vi "Stoic_Mean_Calc-Test.vi"() -> ()   [LabVIEW 2014]
uses:
  <vilib>/Analysis/baseanly.llb/Mean (DBL).vi
  <vilib>/Utility/file.llb/Read From Spreadsheet File (DBL).vi
  <vilib>/Analysis/NI_AALBase.lvlib
panel:
  out "Max":dbl format="%0.2f"
  out "Max Array":dbl[](array[numeric])
  in  "Test Vi":bool
  out "Mean":dbl format="%0.2f"
  out "Mean Array":dbl[](array[numeric])
  out "Min value":dbl
  out "Max value":dbl
  in  "Cycle Length":dbl
  out "20% Bin Index":i32[](array[numeric])
  out "Bin Array":dbl[](array[numeric])
  out "Temp Values":dbl[](array[numeric])
  in  "file path (dialog if empty)":path
  out "Max Bin":dbl
  out "Min Bin":dbl
  in  "Multiple":dbl
  in  "Array In":dbl[](array[numeric])
  # "Stoic Temperature Mean"
  # "Overall"
  # "Stoic"
  # "(Used for Testing)"
  # "For Testing VI:\nUse Tab delimited file from excel with all data Transposed\nto the top Row.\nOpen Vi in Windows not RT."
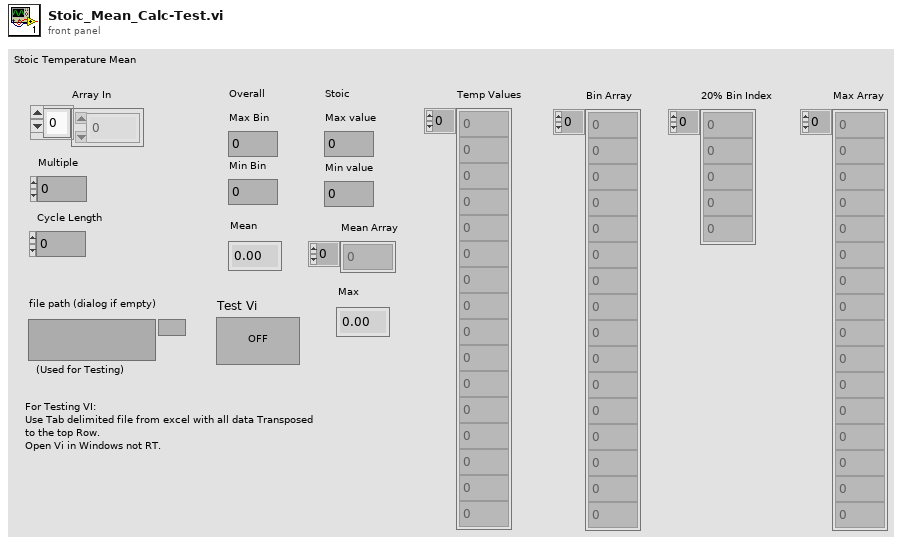
[diagram p1: front panel]
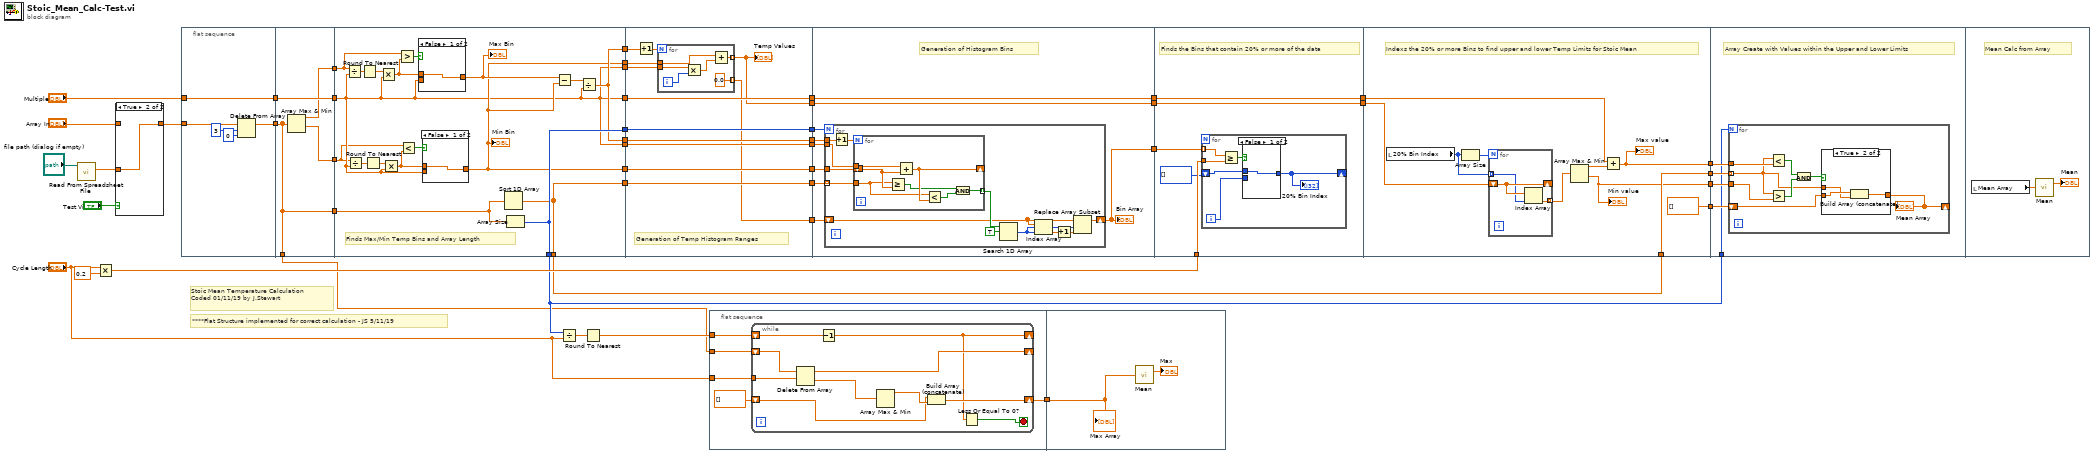
[diagram p0: block diagram]
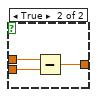
[diagram p3: hidden frame]
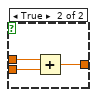
[diagram p4: hidden frame]
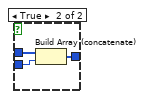
[diagram p5: hidden frame]
diagram:
  # "****Flat Structure implemented for correct calculation - JS 5/11/19"
  # "Stoic Mean Temperature Calculation\nCoded 01/11/19 by J.Stewart"
  n1 = call-poly <vilib>:"Read From Spreadsheet File.vi"("file path (dialog if empty)"="file path (dialog if empty)") -> ("first row"=w45:dbl[])  [unwired: 6 in, 4 out]
  n2 = Multiply(x="Cycle Length", y=0.2) -> (x*y=w38:dbl)
  n3 = case shown="True" "Test Vi" {
    tunnel: w45 -> [_ w49]
    tunnel: [w48 w49] -> w7
    tunnel: "Array In" -> [w48 _]
    frame False {
    }
    frame True {
    }
  }
  n4 = flat-sequence {
    tunnel: "Multiple" -> [w54]
    tunnel: [w54] -> w9
    tunnel: [w51] -> w8
    tunnel: w7 -> [w50]
    tunnel: [w58] -> w13
    tunnel: [w55] -> w12
    tunnel: [w57] -> w11
    tunnel: [w56] -> w10
    tunnel: w9 -> [w58]
    tunnel: w8 -> [w55]
    tunnel: [w55] -> w1
    tunnel: [w74] -> w23
    tunnel: [w65] -> w22
    tunnel: [w60] -> w21
    tunnel: [w73] -> w20
    tunnel: [w75] -> w19
    tunnel: [w60] -> w18
    tunnel: [w73] -> w17
    tunnel: [w65] -> w16
    tunnel: [w75] -> w3
    tunnel: [w74] -> w15
    tunnel: [w60] -> w14
    tunnel: w13 -> [w60]
    tunnel: w12 -> [w76]
    tunnel: w11 -> [w66]
    tunnel: w10 -> [w59]
    tunnel: [w89] -> w36
    tunnel: [w96] -> w35
    tunnel: [w95] -> w34
    tunnel: [w94] -> w33
    tunnel: [w93] -> w32
    tunnel: [w92] -> w31
    tunnel: [w85] -> w29
    tunnel: [w91] -> w26
    tunnel: w23 -> [w96]
    tunnel: w22 -> [w95]
    tunnel: w21 -> [w94]
    tunnel: w20 -> [w93]
    tunnel: w19 -> [w92]
    tunnel: w18 -> [w91]
    tunnel: w17 -> [w88]
    tunnel: w16 -> [w86]
    tunnel: w14 -> [w87]
    tunnel: [w111] -> w37
    tunnel: w36 -> [w110]
    tunnel: w35 -> [w109]
    tunnel: w34 -> [w108]
    tunnel: w33 -> [w107]
    tunnel: w32 -> [w106]
    tunnel: w31 -> [w105]
    tunnel: w29 -> [w104]
    tunnel: [w104] -> w28
    tunnel: w26 -> [w103]
    tunnel: [w103] -> w25
    tunnel: w38 -> [w134]
    tunnel: w37 -> [w135]
    tunnel: [w132] -> w30
    tunnel: w28 -> [w132]
    tunnel: [w131] -> w27
    tunnel: w25 -> [w131]
    tunnel: w15 -> [w155]
    tunnel: [w150] -> w42
    tunnel: [dbl[] [] ("Array 3")] -> w41
    tunnel: [w155] -> w40
    tunnel: [w149] -> w39
    tunnel: w30 -> [w147]
    tunnel: w27 -> [w146]
    tunnel: w42 -> [w162]
    tunnel: w41 -> [w161]
    tunnel: w40 -> [w160]
    tunnel: w39 -> [w163]
    tunnel: w3 -> [w159]
    frame #0 {
      n5 = Delete From Array(array=w50, length=3, index=0) -> (array with subset deleted=w51:dbl[])  [unwired: 1 out]
    }
    frame #1 {
      n6 = Array Max & Min(array=w55) -> (max value=w57:dbl, min value=w56:dbl)  [unwired: 2 out]
    }
    frame #2 {
      # "Finds Max/Min Temp Bins and Array Length"
      n7 = Divide(x=w66, y=w60) -> (x/y=w67:dbl)
      n8 = Divide(x=w59, y=w60) -> (x/y=w61:dbl)
      n9 = Round To Nearest(number=w67) -> (nearest integer value=w68:dbl)
      n10 = Round To Nearest(number=w61) -> (nearest integer value=w62:dbl)
      n11 = Multiply(x=w68, y=w60) -> (x*y=w69:dbl)
      n12 = Multiply(x=w62, y=w60) -> (x*y=w63:dbl)
      n13 = Greater?(x=w66, y=w69) -> (0:w70:bool)
      n14 = Less?(x=w59, y=w63) -> (x < y?=w64:bool)
      n15 = case shown="False" w70 {
        tunnel: w69 -> [w81 w84]
        tunnel: w60 -> [_ w83]
        tunnel: [w81 w82] -> w71
        frame False {
        }
        frame True {
          n16 = Add(x=w84, y=w83) -> (x+y=w82:dbl)
        }
      }
      "Max Bin" <- w71
      n17 = case shown="False" w64 {
        tunnel: w63 -> [w77 w80]
        tunnel: w60 -> [_ w79]
        tunnel: [w77 w78] -> w65
        frame False {
        }
        frame True {
          n18 = Subtract(x=w80, y=w79) -> (x-y=w78:dbl)
        }
      }
      "Min Bin" <- w65
      n19 = Sort 1D Array(array=w76) -> (sorted array=w74:dbl[])
      n20 = Array Size(array=w76) -> (size(s)=w75:i32)
      n21 = Subtract(x=w71, y=w65) -> (x-y=w72:dbl)
      n22 = Divide(x=w72, y=w60) -> (x/y=w73:dbl)
    }
    frame #3 {
      # "Generation of Temp Histogram Ranges"
      n23 = Increment(x=w88) -> (x+1=w90:dbl)
      n24 = for {
        N: w90 -> [_]
        tunnel: w87 -> [w102]
        tunnel: w86 -> [w101]
        tunnel: [w99] -> w85 mode=indexing
        tunnel: [0.0 ("x+y")] -> w89 mode=indexing
        i -> [w98]
        n25 = Multiply(x=w102, y=w98) -> (x*y=w100:dbl)
        n26 = Add(x=w101, y=w100) -> (x+y=w99:dbl)
      }
      "Temp Values" <- w85
    }
    frame #4 {
      # "Generation of Histogram Bins"
      n27 = for {
        N: w105 -> [_]
        tunnel: w107 -> [w122]
        tunnel: w109 -> [w123] mode=indexing
        tunnel: w106 -> [w112]
        tunnel: w108 -> [w121]
        shift-right: [w120] -> w111
        shift-left: w110 -> [w116]
        n28 = Increment(x=w112) -> (x+1=w113:dbl)
        n29 = for {
          N: w113 -> [_]
          tunnel: w123 -> [w126]
          tunnel: w122 -> [w124]
          shift-right: [w129] -> _
          shift-left: w121 -> [w130]
          tunnel: [w125] -> w119 mode=indexing
          n30 = Greater Or Equal?(x=w126, y=w130) -> (x >= y?=w127:bool)
          n31 = Add(x=w124, y=w130) -> (x+y=w129:dbl)
          n32 = Less?(x=w126, y=w129) -> (x < y?=w128:bool)
          n33 = And(x=w127, y=w128) -> (x .and. y?=w125:bool)
        }
        n34 = Search 1D Array(1D array=w119, element=TRUE) -> (index of element=w117:i32)  [unwired: 1 in]
        n35 = Index Array(array=w116, index=w117) -> (element=w115:dbl)
        n36 = Increment(x=w115) -> (x+1=w114:dbl)
        n37 = Replace Array Subset(array=w116, new element=w114, index=w117) -> (w120:dbl[])
      }
      "Bin Array" <- w111
    }
    frame #5 {
      # "Finds the Bins that contain 20% or more of the data"
      n38 = for {
        tunnel: w135 -> [w141] mode=indexing
        shift-right: [w138] -> _
        shift-left: i32[] [] -> [w137]
        tunnel: w134 -> [w136]
        i -> [w139]
        n39 = Greater Or Equal?(x=w141, y=w136) -> (x >= y?=w140:bool)
        n40 = case shown="False" w140 {
          tunnel: w139 -> [_ w145]
          tunnel: [w142 w144] -> w138
          tunnel: w137 -> [w142 w143]
          frame False {
          }
          frame True {
            n41 = Build Array (concatenate)(w143, w145) -> (w144:i32[])
          }
        }
        "20% Bin Index" <- w138
      }
    }
    frame #6 {
      # "Indexs the 20% or more Bins to find upper and lower Temp Limits for Stoic Mean"
      n42 = local read "20% Bin Index"() -> (w148:i32[])
      n43 = Array Size(array=w148) -> (size(s)=w151:i32)
      n44 = for {
        N: w151 -> [_]
        tunnel: w148 -> [w157] mode=indexing
        shift-right: [w158] -> _
        shift-left: w147 -> [w158]
        tunnel: [w156] -> w152 mode=indexing
        n45 = Index Array(array=w158, index=w157) -> (element=w156:dbl)
      }
      n46 = Array Max & Min(array=w152) -> (max value=w153:dbl, min value=w149:dbl)  [unwired: 2 out]
      "Min value" <- w149
      n47 = Add(x=w146, y=w153) -> (x+y=w150:dbl)
      "Max value" <- w150
    }
    frame #7 {
      # "Array Create with Values within the Upper and Lower Limits"
      n48 = for {
        N: w159 -> [_]
        tunnel: w163 -> [w171]
        tunnel: w162 -> [w170]
        shift-right: [w164] -> _
        shift-left: w161 -> [w166]
        tunnel: w160 -> [w165] mode=indexing
        n49 = Less?(x=w165, y=w170) -> (x < y?=w169:bool)
        n50 = Greater?(x=w165, y=w171) -> (0:w168:bool)
        n51 = And(x=w169, y=w168) -> (x .and. y?=w167:bool)
        n52 = case shown="True" w167 {
          tunnel: w166 -> [w172 w175]
          tunnel: [w172 w174] -> w164
          tunnel: w165 -> [_ w173]
          frame False {
          }
          frame True {
            n53 = Build Array (concatenate)(w175, w173) -> (w174:dbl[])
          }
        }
        "Mean Array" <- w164
      }
    }
    frame #8 {
      # "Mean Calc from Array"
      n54 = local read "Mean Array"() -> (w177:dbl[])
      n55 = call-poly <vilib>:"Mean.vi"("X"=w177) -> ("mean"=→"Mean":dbl)  [unwired: 1 out]
    }
  }
  n56 = Divide(x=w3, y="Cycle Length") -> (x/y=w4:dbl)
  n57 = Round To Nearest(number=w4) -> (nearest integer value=w5:dbl)
  n58 = flat-sequence {
    tunnel: w1 -> [w182]
    tunnel: w5 -> [w181]
    tunnel: "Cycle Length" -> [w180]
    tunnel: [w178] -> w6
    tunnel: w6 -> [w193]
    frame #0 {
      n59 = while {
        shift-right: [w190] -> _
        shift-left: w182 -> [w192]
        tunnel: w180 -> [w191]
        shift-right: [w188] -> w178
        shift-left: dbl[] [] -> [w186]
        shift-right: [w183] -> _
        shift-left: w181 -> [w185]
        stop <- w184 stop-if-true
        n60 = Delete From Array(array=w192, length=w191) -> (deleted portion=w189:dbl[], array with subset deleted=w190:dbl[])  [unwired: 1 in]
        n61 = Decrement(x=w185) -> (x-1=w183:dbl)
        n62 = Array Max & Min(array=w189) -> (max value=w187:dbl)  [unwired: 3 out]
        n63 = Build Array (concatenate)(w186, w187) -> (w188:dbl[])
        n64 = Less Or Equal To 0?(x=w183) -> (x <= 0?=w184:bool)
      }
    }
    frame #1 {
      n65 = call-poly <vilib>:"Mean.vi"("X"=w193) -> ("mean"=→"Max":dbl)  [unwired: 1 out]
      "Max Array" <- w193
    }
  }
